vi "Start Data Logger.vi"(8 "error in (no error)":errorcluster, 9 "Trigger Source (0: Bus)":i32(ring) items=["Bus", "External", "Immediate"], 10 "Data Save Path (\"External:\\log_1.csv\")":string="\"External:\\log_1.csv\"", 11 "VISA resource name":refnum<visa-resource-name>) -> (0 "error out":errorcluster, 3 "VISA resource name out":refnum<visa-resource-name>)   [LabVIEW 2020, in "Keysight E36300 Series.lvlib"]
doc: "Starts the internal data logging session.\n\n<b>Note: </b>\nThis VI is only applicable for E36312A and E36313A models."
uses:
  Keysight E36300 Series.lvlib
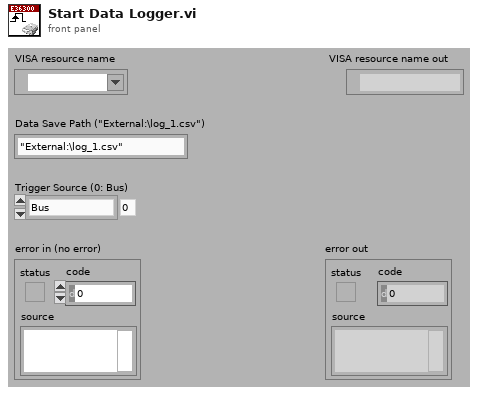
[diagram p1: front panel]
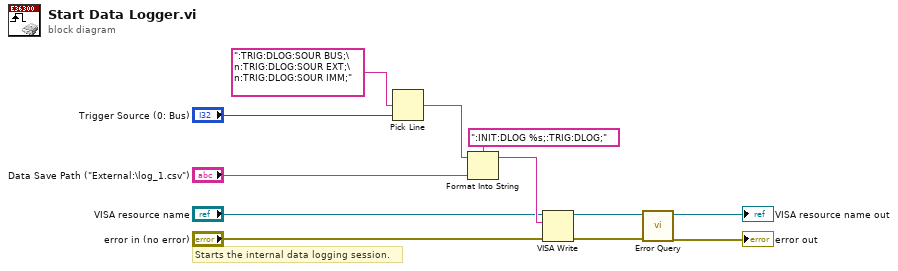
[diagram p0: block diagram]
diagram:
  # "Starts the internal data logging session."
  n1 = Pick Line(multi-line string=":TRIG:DLOG:SOUR BUS;\n:TRIG:DLOG:SOUR EXT;\n:TRIG:DLOG:SOUR IMM;", line index="Trigger Source (0: Bus)") -> (output string=w10:string)  [unwired: 1 in]
  n2 = Format Into String(format string=":INIT:DLOG %s;:TRIG:DLOG;", initial string=w10, "Data Save Path (\"External:\\log_1.csv\")") -> (resulting string=w7:string)  [unwired: 1 in, 1 out]
  n3 = VISA Write(VISA resource name="VISA resource name", write buffer=w7, error in (no error)="error in (no error)") -> (VISA resource name out=w4:refnum<visa-resource-name>, error out=w3:errorcluster)  [unwired: 1 out]
  n4 = call "Error Query.vi"("error in (no error)"=w3, "VISA resource name"=w4) -> ("error out"=→"error out":errorcluster, "VISA resource name out"=→"VISA resource name out":refnum<visa-resource-name>)  [unwired: 6 in, 2 out]
